vi "read_n_neighbors.vi"(8 "error in (no error)":errorcluster, 11 "KNeighbors in":refnum<class "KNeighbors.lvclass">) -> (0 "error out":errorcluster, 2 "n_neighbors":dbl, 3 "KNeighbors out":refnum<class "KNeighbors.lvclass">)   [LabVIEW 2020, in "KNeighbors.lvclass"]
uses:
  KNeighbors.lvclass
  KNeighbors.lvclass/KNeighbors.ctl
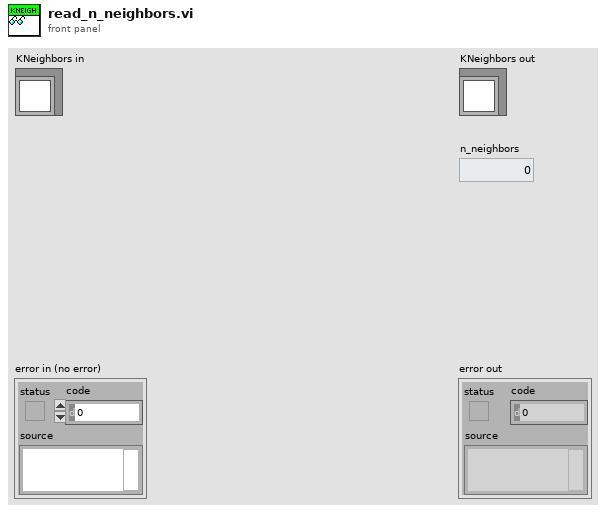
[diagram p1: front panel]
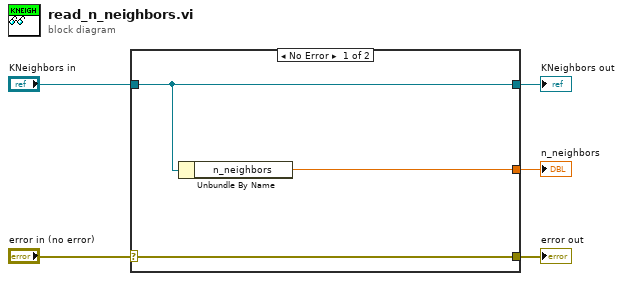
[diagram p0: block diagram]
diagram:
  n1 = case shown="No Error" "error in (no error)" {
    selector: "error in (no error)" -> [w8 w9]
    tunnel: [w8 w9] -> w4
    tunnel: [w7 w10] -> w2
    tunnel: "KNeighbors in" -> [w7 w10]
    tunnel: [w6 _] -> w1
    frame No Error {
      n2 = Unbundle By Name(w7) -> ("n_neighbors"=w6:dbl)
    }
    frame Error {
    }
  }
  "error out" <- w4
  "KNeighbors out" <- w2
  "n_neighbors" <- w1
